vi "강도플롯.vi"() -> ()   [LabVIEW 2014]
panel:
  out "강도 그래프 2":dbl[][](graph)
  out "강도 그래프":dbl[][](graph)
  out "배열":dbl[][](array[numeric])
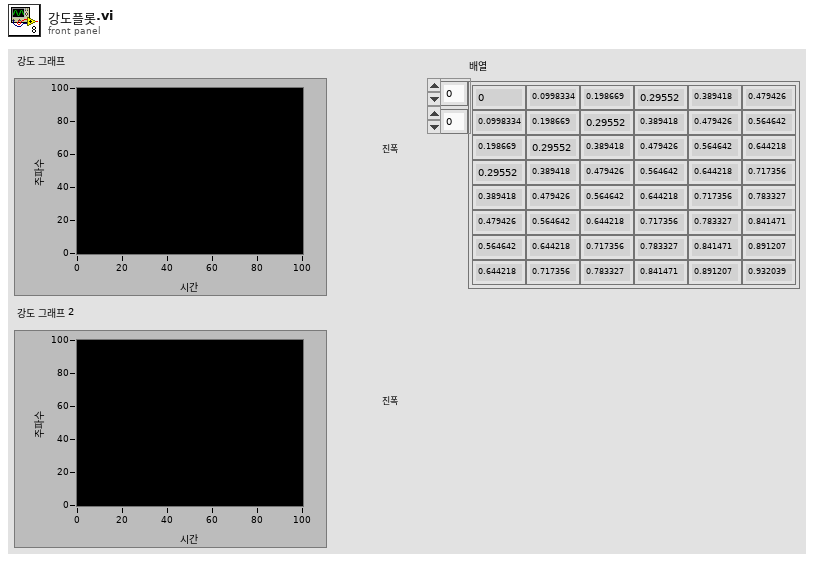
[diagram p1: front panel]
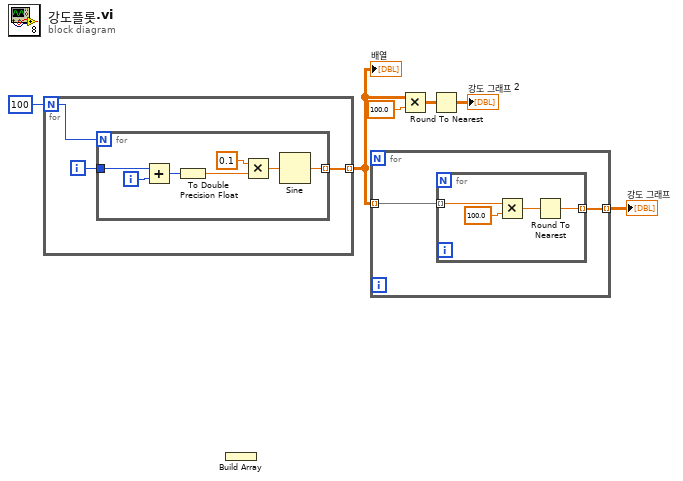
[diagram p0: block diagram]
diagram:
  n1 = for {
    N: 100 -> [w9]
    tunnel: [w7] -> w4 mode=indexing
    i -> [w8]
    n2 = for {
      N: w9 -> [_]
      tunnel: w8 -> [w16]
      tunnel: [w10] -> w7 mode=indexing
      i -> [w15]
      n3 = Add(x=w16, y=w15) -> (x+y=w14:i32)
      n4 = To Double Precision Float(number=w14) -> (double precision float=w13:dbl)
      n5 = Multiply(x=0.1, y=w13) -> (x*y=w11:dbl)
      n6 = Sine(x=w11) -> (sin(x)=w10:dbl)
    }
  }
  "배열" <- w4
  n7 = Build Array() -> ()  [unwired: 1 in, 1 out]
  n8 = for {
    tunnel: w4 -> [w18] mode=indexing
    tunnel: [w17] -> w5 mode=indexing
    n9 = for {
      tunnel: w18 -> [w22] mode=indexing
      tunnel: [w19] -> w17 mode=indexing
      n10 = Multiply(x=w22, y=100.0) -> (x*y=w20:dbl)
      n11 = Round To Nearest(number=w20) -> (nearest integer value=w19:dbl)
    }
  }
  "강도 그래프" <- w5
  n12 = Multiply(x=w4, y=100.0) -> (x*y=w2:dbl[][])
  n13 = Round To Nearest(number=w2) -> (nearest integer value=→"강도 그래프 2":dbl[][])
